vi "LS218_ConfigSerial.vi"(5 "error in":errorcluster, 8 "VISA":refnum<visa-resource-name>) -> (0 "error out":errorcluster, 2 "ID String":string, 3 "VISA Out":refnum<visa-resource-name>)   [LabVIEW 2012, in "Lake Shore Cryotronics 218.lvlib"]
doc: "This VI passes the COM PORT to the VISA Config Serial VI and returns the instrument ID. \nIt reads ID back to test if the initialisation is successful. \n\nCall this before using any of the instrument driver VIs for this instrument.\n\n\nHARPS-N use"
uses:
  <instrlib>/Lake Shore Cryotronics 218/Lake Shore Cryotronics 218.lvlib
  <vilib>/Instr/_visa.llb/VISA Configure Serial Port (Instr).vi
panel:
  # "for HARPS-N use"
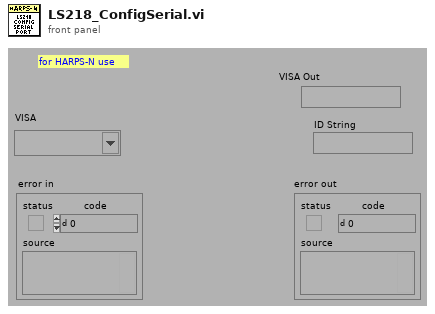
[diagram p1: front panel]
types:
  T1 = cluster{"Timeout Value (10000)":u32, "Baud Rate (57600)":enum16{"1200", "2400", "4800", "9600", "19200", "38400", "57600", "115200"}, "Flow Control (1:XON/XOFF)":enum16{"None", "XON / XOFF", "RTS / CTS", "DTR / DSR"}}
  T2 = enum16{"1200", "2400", "4800", "9600", "19200", "38400", "57600", "115200"}
  T3 = enum16{"None", "XON / XOFF", "RTS / CTS", "DTR / DSR"}
  T4 = cluster{"Status":bool, "Code":i32, "Source (VI Name)":string}
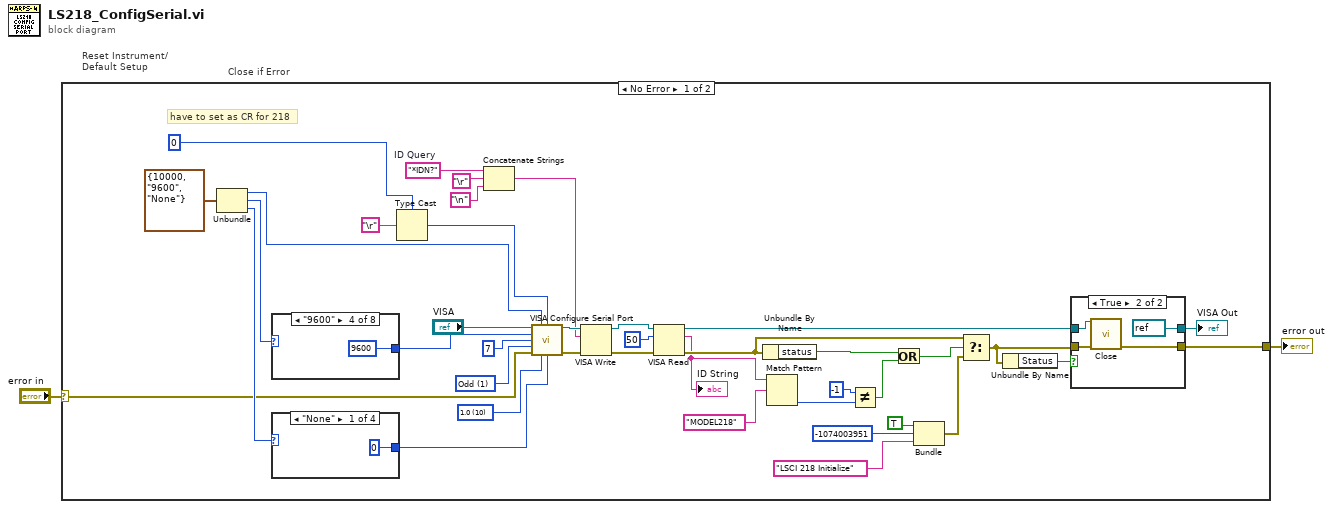
[diagram p0: block diagram]
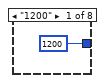
[diagram p3: hidden frame]
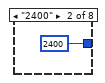
[diagram p4: hidden frame]
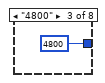
[diagram p5: hidden frame]
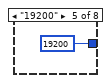
[diagram p6: hidden frame]
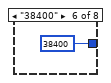
[diagram p7: hidden frame]
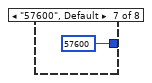
[diagram p8: hidden frame]
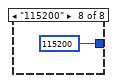
[diagram p9: hidden frame]
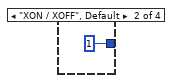
[diagram p10: hidden frame]
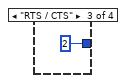
[diagram p11: hidden frame]
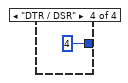
[diagram p12: hidden frame]
diagram:
  # "Close if Error"
  # "Reset Instrument/\nDefault Setup"
  n1 = case shown="No Error" "error in" {
    selector: "error in" -> [w30 w61]
    tunnel: [w11 w61] -> w1
    frame No Error {
      w6 = "*IDN?"  # ID Query
      w41 = u16 10 items=["1.0"=10, "1.5"=15, "2.0"=20] ("Serial Settings:Stop Bits")
      w40 = u16 1 items=["None", "Odd", "Even", "Mark", "Space"] ("Serial Settings:Serial Parity")
      # "have to set as CR for 218"
      n2 = Unbundle(T1 {"Timeout Value (10000)"=10000, "Baud Rate (57600)"=enum."9600", "Flow Control (1:XON/XOFF)"=enum."None"} ("Serial Port Configuration")) -> ("Timeout Value (10000)"=w38:u32, "Baud Rate (57600)"=w34:T2, "Flow Control (1:XON/XOFF)"=w35:T3)
      n3 = case shown="\"9600\"" w34 {
        tunnel: [u32 1200 u32 2400 u32 4800 u32 9600 u32 19200 u32 38400 u32 57600 u32 115200] -> w37
        frame "1200" {
        }
        frame "2400" {
        }
        frame "4800" {
        }
        frame "9600" {
        }
        frame "19200" {
        }
        frame "38400" {
        }
        frame "57600", Default {
        }
        frame "115200" {
        }
      }
      n4 = case shown="\"None\"" w35 {
        tunnel: [u16 0 u16 1 u16 2 u16 4] -> w36
        frame "None" {
        }
        frame "XON / XOFF", Default {
        }
        frame "RTS / CTS" {
        }
        frame "DTR / DSR" {
        }
      }
      n5 = Type Cast(type=u8 0, x="\r") -> (*(type *) &x=w31:u8)
      n6 = Concatenate Strings(w6, "\r", "\n") -> (w4:string)
      n7 = call-poly "VISA Configure Serial Port"("VISA resource name"="VISA", "timeout (10sec)"=w38, "termination char\n(0xA = '\\n' = LF)"=w31, "baud rate (9600)"=w37, "data bits (8)"=u16 7 ("Serial Settings:Serial Data Bits"), "parity (0:none)"=w40, "error in (no error)"=w30, "stop bits (10: 1 bit)"=w41, "flow control (0:none)"=w36) -> ("VISA resource name out"=w10:refnum<visa-resource-name>, "error out"=w14:errorcluster)  [unwired: 5 in]
      n8 = VISA Write(VISA resource name=w10, write buffer=w4, error in (no error)=w14) -> (VISA resource name out=w18:refnum<visa-resource-name>, error out=w20:errorcluster)  [unwired: 1 out]
      n9 = VISA Read(VISA resource name=w18, byte count=u32 50, error in (no error)=w20) -> (VISA resource name out=w9:refnum<visa-resource-name>, read buffer=w17:string, error out=w19:errorcluster)  [unwired: 1 out]
      "ID String" <- w17
      n10 = Unbundle By Name(w19) -> ("status"=w22:bool)
      n11 = Match Pattern(string=w17, regular expression="MODEL218") -> (offset past match=w25:i32)  [unwired: 1 in, 3 out]
      n12 = Not Equal?(x=-1, y=w25) -> (x != y?=w16:bool)
      n13 = Or(x=w22, y=w16) -> (x .or. y?=w21:bool)
      n14 = Bundle("Status"=TRUE, "Code"=-1074003951, "Source (VI Name)"="LSCI 218 Initialize") -> (w27:T4)  [unwired: 1 in]
      n15 = Select(t=w19, s=w21, f=w27) -> (s? t:f=w12:T4)
      n16 = Unbundle By Name(w12) -> ("Status"=w8:bool)
      n17 = case shown="True" w8 {
        tunnel: [w43 refnum<visa-resource-name> refnum ("VISA resource name out")] -> w13
        tunnel: [w44 w48] -> w11
        tunnel: w12 -> [w44 w46]
        tunnel: w9 -> [w43 w45]
        frame False {
        }
        frame True {
          n18 = call <instrlib>:"Close.vi"("VISA resource name"=w45, "error in (no error)"=w46) -> ("error out"=w48:errorcluster)  [unwired: 13 in]
        }
      }
      "VISA Out" <- w13
    }
    frame Error {
    }
  }
  "error out" <- w1
